vi "Set Module Config.vi"(8 "error in (no error)":errorcluster, 10 "Config Channels":dbl[](array[numeric]), 11 "9237 in":refnum<class "9237.lvclass">) -> (0 "error out":errorcluster, 3 "9237 out":refnum<class "9237.lvclass">)   [LabVIEW 2011, in "Modules.lvlib" / "9237.lvclass"]
uses:
  9237.lvclass
  9237.lvclass/9237.ctl
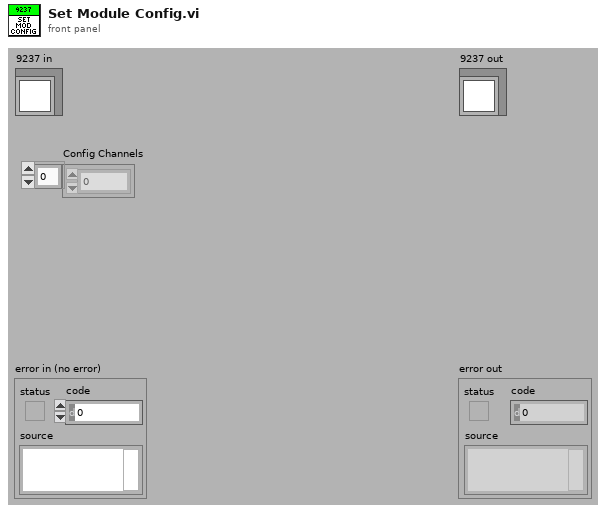
[diagram p1: front panel]
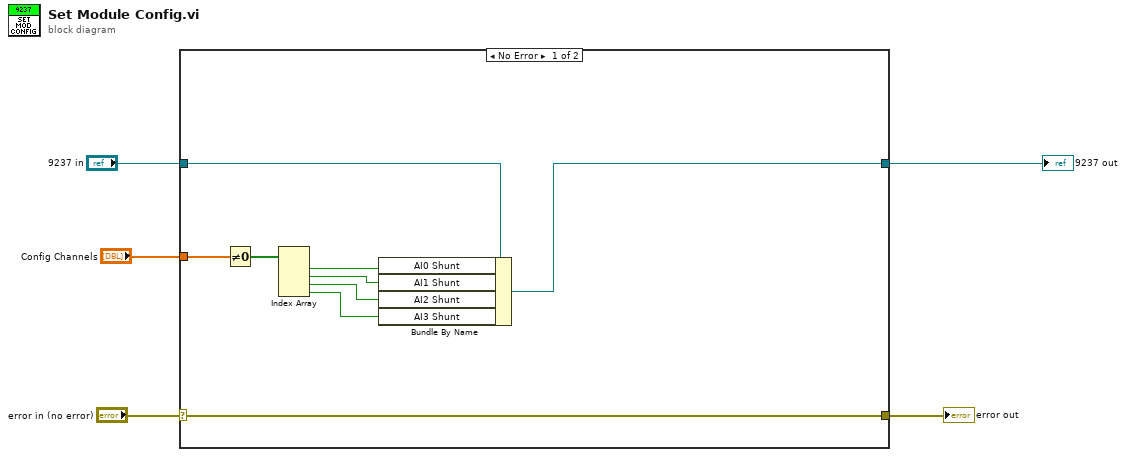
[diagram p0: block diagram]
diagram:
  n1 = case shown="No Error" "error in (no error)" {
    selector: "error in (no error)" -> [w6 w16]
    tunnel: "9237 in" -> [w14 w15]
    tunnel: "Config Channels" -> [w13 _]
    tunnel: [w6 w16] -> w2
    tunnel: [w7 w15] -> w1
    frame No Error {
      n2 = Not Equal To 0?(x=w13) -> (x != 0?=w12:bool[])
      n3 = Index Array(array=w12) -> (element #1=w11:bool, element #2=w10:bool, element #3=w9:bool, element #4=w8:bool)  [unwired: 4 in]
      n4 = Bundle By Name(cluster=w14, "AI0 Shunt"=w11, "AI1 Shunt"=w10, "AI2 Shunt"=w9, "AI3 Shunt"=w8) -> (w7:refnum<class "9237.lvclass">)
    }
    frame Error {
    }
  }
  "error out" <- w2
  "9237 out" <- w1
